vi "email client log.vi"(8 "error in":errorcluster) -> (0 "error out":errorcluster)   [LabVIEW 2012]
uses:
  ReadWrite.ctl
  Design Server.lvlib
panel:
  out "date string":string
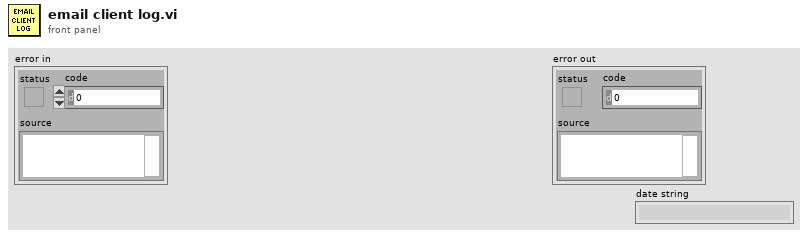
[diagram p1: front panel]
types:
  T1 = typedef "ReadWrite.ctl" = enum16{"Read", "Write"}
  T2 = enum16{"open", "replace", "create", "open or create", "replace or create", "replace or create with confirmation"}
  T3 = typedef "Mail Server.ctl" = cluster{"Outgoing Mail Server (SMTP)":string, "MAIL Account User ID":string, "MAIL Account Password":string, "Enable SSL":bool, "Port":i32, "Sender's Email Address":string, "Sender's Name":string}
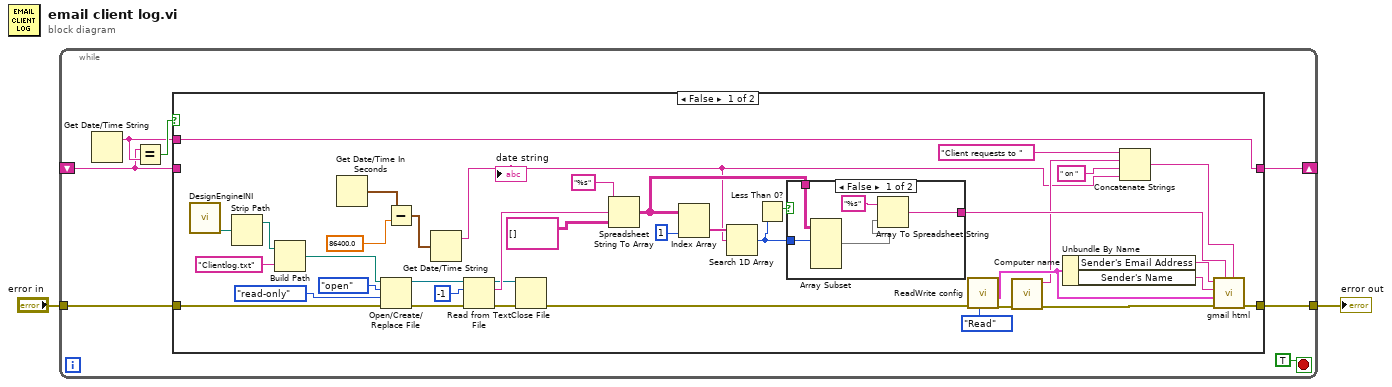
[diagram p0: block diagram]
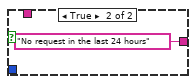
[diagram p2: hidden frame]
diagram:
  n1 = while {
    shift-right: [w9] -> _
    shift-left: _ -> [w6]
    tunnel: [w4] -> w2
    tunnel: "error in" -> [w3]
    stop <- TRUE stop-if-true
    n2 = Get Date/Time String() -> (date string=w7:string)  [unwired: 3 in, 1 out]
    n3 = Equal?(x=w6, y=w7) -> (x = y?=w8:bool)
    n4 = case shown="False" w8 {
      tunnel: [w47 w55] -> w9
      tunnel: w7 -> [w47 _]
      tunnel: w6 -> [_ w55]
      tunnel: [w17 w54] -> w4
      tunnel: w3 -> [w16 w54]
      frame False {
        n5 = call "DesignEngineINI.vi"() -> ("Ini file path"=w45:path)  [unwired: 6 in, 1 out]
        n6 = Strip Path(path=w45) -> (stripped path=w44:path)  [unwired: 1 out]
        n7 = Build Path(base path=w44, name or relative path="Clientlog.txt") -> (appended path=w43:path)
        n8 = Get Date/Time In Seconds() -> (seconds since 1Jan1904=w14:timestamp)
        n9 = Open/Create/Replace File(file path (use dialog)=w43, error in=w16, operation (0:open)=T2."open", access (0:read/write)=enum16{"read/write", "read-only", "write-only"}."read-only") -> (refnum out=w38:refnum<file>, error out=w40:errorcluster)  [unwired: 2 in, 1 out]
        n10 = Subtract(x=w14, y=86400.0 ("x-y")) -> (x-y=w13:timestamp)
        n11 = Get Date/Time String(seconds (now)=w13) -> (date string=w12:string)  [unwired: 2 in, 1 out]
        "date string" <- w12
        n12 = Read from Text File(file (use dialog)=w38, count=-1, error in=w40) -> (refnum out=w35:refnum<file>, text=w39:string, error out=w34:errorcluster)  [unwired: 1 in, 1 out]
        n13 = Close File(refnum=w35, error in=w34) -> (error out=w28:errorcluster)  [unwired: 1 out]
        n14 = Spreadsheet String To Array(format string="%s", spreadsheet string=w39, array type (2D Dbl)=string[][] [] ("Array")) -> (array=w30:string[][])  [unwired: 1 in]
        n15 = Index Array(array=w30, index (col)=1 ("disabled index (col)")) -> (element=w31:string[])  [unwired: 1 in]
        n16 = Search 1D Array(1D array=w31, element=w12) -> (index of element=w11:i32)  [unwired: 1 in]
        n17 = Less Than 0?(x=w11) -> (x < 0?=w10:bool)
        n18 = case shown="False" w10 {
          tunnel: w30 -> [w52 _]
          tunnel: w11 -> [w51 _]
          tunnel: [w48 "No request in the last 24 hours" ("spreadsheet string")] -> w29
          frame False {
            n19 = Array Subset(array=w52, index (row)=w51) -> (w50:string[][])  [unwired: 3 in]
            n20 = Array To Spreadsheet String(array=w50, 3:"%s" ("format string")) -> (spreadsheet string=w48:string)  [unwired: 1 in]
          }
          frame True {
          }
        }
        n21 = call "ReadWrite config.vi"("Config"=ReadWrite."Read", "error in (no error)"=w28) -> ("error out"=w19:errorcluster, "Mail Server"=w26:T3)  [unwired: 6 in, 2 out]
        n22 = call "Computer name.vi"("error in (no error)"=w19) -> ("error out"=w18:errorcluster, "Computer web address"=w23:string)  [unwired: 8 in, 1 out]
        n23 = Unbundle By Name(w26) -> ("Sender's Email Address"=w25:string, "Sender's Name"=w24:string)
        n24 = Concatenate Strings("Client requests to " ("string"), w23, " on " ("string"), w12) -> (w20:string)
        n25 = call "gmail html.vi"("Subject"=w20, "Body"=w29, "error in (no error)"=w18, "Server"=w26, "Recipient's Name"=w24, "Recipient's Email Address"=w25) -> ("error out"=w17:errorcluster)  [unwired: 5 in]
      }
      frame True {
        # "date hasn't changed since the last time it sent a message"
      }
    }
  }
  "error out" <- w2
